vi "All Sensors.vi"() -> ()   [LabVIEW 2019]
uses:
  <vilib>/Platform/TimedLoop/XDataNode/timing_clust.ctl
  <vilib>/Platform/TimedLoop/XDataNode/nitl_modes.ctl
  <vilib>/Platform/TimedLoop/XDataNode/wakeup.ctl
  <vilib>/myRIO/Instrument Drivers/Onboard IO/I2C/typedefs/I2C User Configuration.ctl
  <vilib>/myRIO/Instrument Drivers/Onboard IO/I2C/typedefs/I2C Transfer Rate.ctl
  <vilib>/myRIO/Instrument Drivers/Onboard IO/I2C/typedefs/I2C Reference.ctl
  <vilib>/myRIO/Common/Instrument Driver Framework/Utilities/typedefs/myRIO Generic Hardware Reference.ctl
  <vilib>/myRIO/Common/Instrument Driver Framework/Utilities/typedefs/Hardware Version Enum.ctl
  <vilib>/myRIO/Common/Instrument Driver Framework/Utilities/typedefs/myRIO v1.0 Reference.ctl
  <vilib>/myRIO/Common/Instrument Driver Framework/Utilities/typedefs/Generic FPGA Reference.ctl
  <vilib>/myRIO/Common/Instrument Driver Framework/myRIO v1.0/I2C/typedefs/I2C Channels Enum.ctl
  <vilib>/myRIO/Instrument Drivers/Onboard IO/I2C/typedefs/I2C Configuration.ctl
  <vilib>/userDefined/High Color/nirio_resource_hc.ctl
  <vilib>/myRIO/Common/Instrument Driver Framework/Utilities/vis/Is FPGA Ref Available.vi
  <vilib>/myRIO/Common/Instrument Driver Framework/myRIO v1.0/I2C/vis/myRIO v1.1 Open I2C.vi
  <vilib>/myRIO/Instrument Drivers/Onboard IO/I2C/vis/Configure.vi
  <vilib>/myRIO/Instrument Drivers/Onboard IO/I2C/vis/Write.vi
  <vilib>/myRIO/Instrument Drivers/Onboard IO/I2C/vis/Write Read.vi
  <vilib>/myRIO/Common/Instrument Driver Framework/Utilities/vis/Validate Channels.vi
  <vilib>/myRIO/Common/Instrument Driver Framework/myRIO v1.0/I2C/vis/myRIO v1.0 Reserve I2C.vi
  <vilib>/myRIO/Common/Instrument Driver Framework/myRIO v1.0/I2C/vis/myRIO v1.0 Build MUX Configuration I2C.vi
  <vilib>/myRIO/Common/Instrument Driver Framework/myRIO v1.0/Resource Manager/vis/myRIO v1.0 Reserve Channel List.vi
  <vilib>/myRIO/Common/Instrument Driver Framework/myRIO v1.0/Resource Manager/vis/myRIO v1.0 Create Configuration List.vi
  <vilib>/myRIO/Common/Instrument Driver Framework/myRIO v1.0/Resource Manager/vis/myRIO v1.0 Reserve Channel.vi
  <vilib>/myRIO/Common/Instrument Driver Framework/myRIO v1.0/Resource Manager/vis/myRIO v1.0 Unreserve Channel.vi
  <vilib>/myRIO/Common/Instrument Driver Framework/myRIO v1.0/Resource Manager/vis/myRIO v1.0 Build Mutex Name.vi
  <vilib>/Utility/VariantDataType/GetNumericInfo.vi
  <vilib>/Utility/error.llb/Error Cluster From Error Code.vi
  <vilib>/myRIO/Common/Instrument Driver Framework/myRIO v1.0/myRIO v1.1 Open.vi
  <vilib>/myRIO/Common/Instrument Driver Framework/Utilities/vis/IO Manager.vi
  <vilib>/myRIO/Common/Instrument Driver Framework/Utilities/vis/Configuration Manager.vi
  <vilib>/myRIO/Common/Instrument Driver Framework/myRIO v1.0/Resource Manager/vis/myRIO v1.0 Configure IO.vi
  <vilib>/myRIO/Common/Instrument Driver Framework/myRIO v1.0/myRIO v1.0 Close.vi
  <vilib>/myRIO/Common/Instrument Driver Framework/myRIO v1.0/I2C/vis/myRIO v1.0 Configure I2C.vi
  <vilib>/myRIO/Common/Instrument Driver Framework/myRIO v1.0/I2C/vis/myRIO v1.0 Write I2C.vi
  <vilib>/myRIO/Common/Instrument Driver Framework/myRIO v1.0/I2C/vis/myRIO v1.0 Read I2C.vi
  <vilib>/platform/TimedLoop/XDataNode/XDataNode.xnode
  <vilib>/myRIO/Express VI/Onboard IO/I2C/I2C Express VI.xnode
  <vilib>/myRIO/Instrument Drivers/Onboard IO/I2C/vis/myRIO I2C Open.xnode
  <vilib>/Platform/TimedLoop/XDataNode/XDNodeRunTimeDep.lvlib
  <vilib>/myRIO/Instrument Drivers/Onboard IO/I2C/I2C.lvlib
panel:
  out "Magnetic field [G] 74-2 2":cluster{dbl, dbl, dbl}(graph) caption="Waveform Chart"
  out "Z_mag 6":dbl
  out "Y_mag 6":dbl
  out "X_mag 6":dbl
  out "Z 6":i16
  out "Y 6":i16
  out "X 6":i16
  out "DATA1 6":u8[](array[numeric]) format="%02x"
  in  "[ESC]":bool
  out "appended array":u8[](array[numeric])
  out "Magnetic field [G] 74-2":cluster{dbl, dbl, dbl}(graph) caption="Waveform Chart"
  out "Z_mag 5":dbl
  out "Y_mag 5":dbl
  out "X_mag 5":dbl
  out "Z 5":i16
  out "Y 5":i16
  out "X 5":i16
  out "DATA1 5":u8[](array[numeric]) format="%02x"
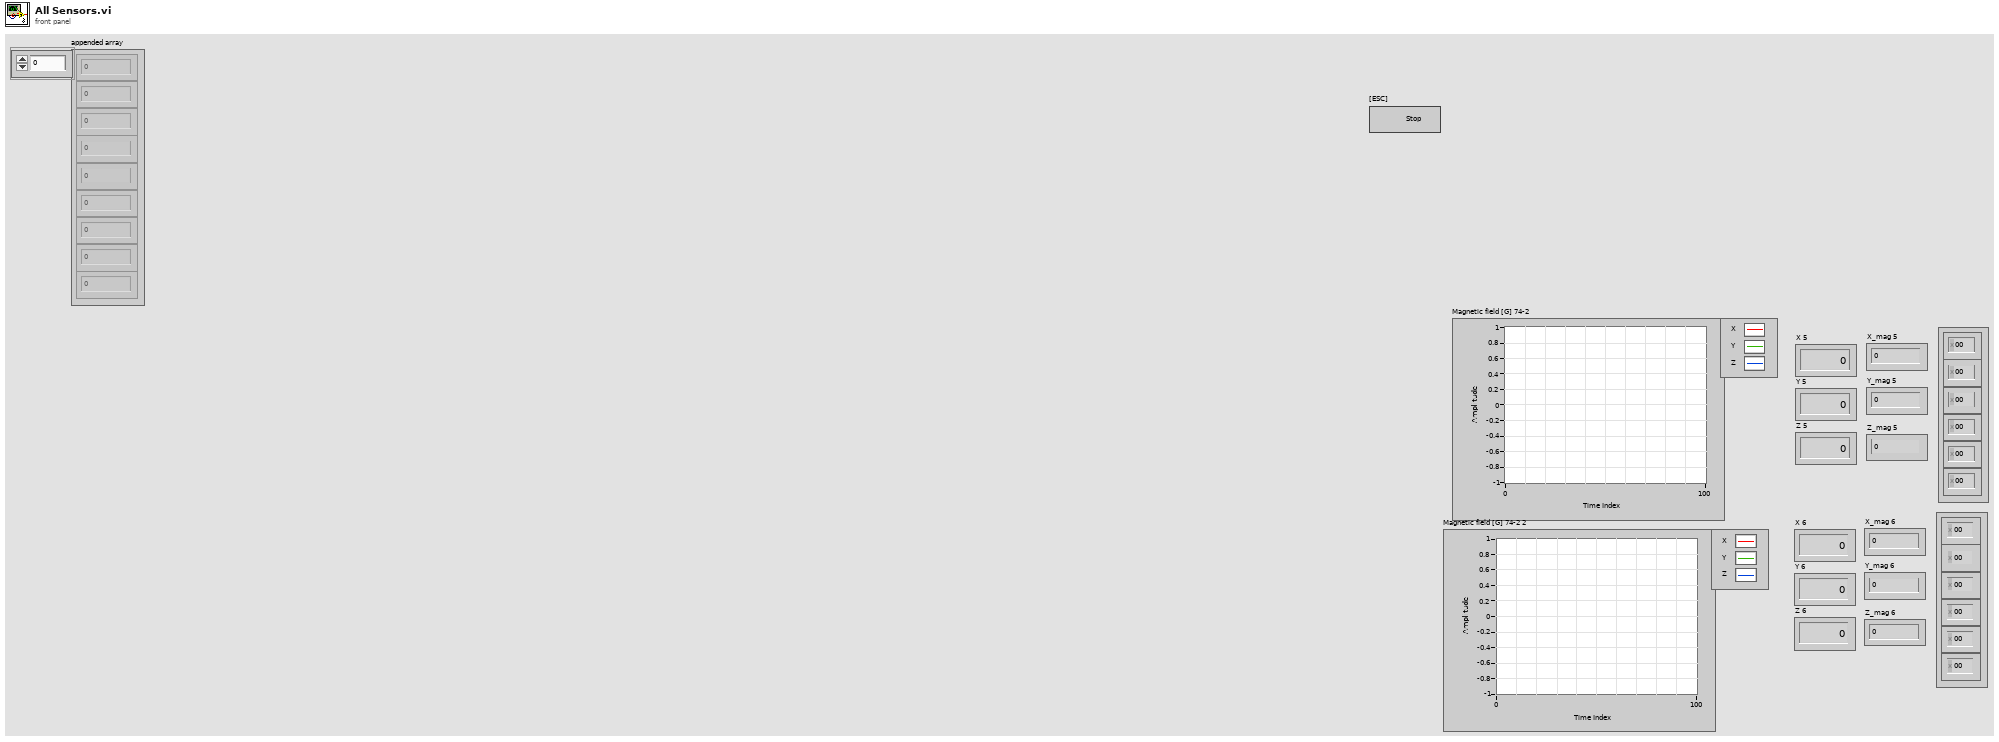
[diagram p1: front panel]
types:
  T1 = typedef "XDNodeRunTimeDep.lvlib/timing_clust.ctl" = cluster{"Expected End [f-1]":u64, "Actual End [f-1]":u64, "Finished Late? [f-1]":bool, "Expected End [i-1]":u64, "Actual End [i-1]":u64, "Finished Late? [i-1]":bool, "Expected Start [i]":u64, "Actual Start [i]":u64, "Expected Start [f]":u64, "Actual Start [f]":u64, "Source Name":string, "Structure Name":string, "Period":i64, "Deadline":i64, "Offset":i64, "Start":i64, "Priority":i32, "Timeout":i32, "Mode":T2, "Wakeup Reason":T3, "Error":errorcluster, "Source Type":string, "Secondary Source Type":string, "Global End Time":u64, "Global Start Time":u64, "Frame Duration":u64, "Iteration Duration":u64, "Assigned CPU":i32, "I/O Scan Engine Mode":u32}
  T2 = typedef "XDNodeRunTimeDep.lvlib/nitl_modes.ctl" = enum32{"No Change", "Process missed periods, maintain original phase", "Discard missed periods, maintain original phase", "Process missed periods, ignore original phase", "Discard missed periods, ignore original phase"}
  T3 = typedef "XDNodeRunTimeDep.lvlib/wakeup.ctl" = enum32{"Normal", "Aborted", "Asynchronous wakeup", "Timing source error", "Timed loop error", "Timeout"}
  T4 = typedef "I2C.lvlib/I2C Reference.ctl" = cluster{"myRIO Reference":T5, "I2C Channels Enum":T9, "I2C Configuration":T10}
  T5 = typedef "myRIO Generic Hardware Reference.ctl" = cluster{"myRIO Model":T6, "myRIO Hardware Reference":T7}
  T6 = typedef "Hardware Version Enum.ctl" = enum16{"Unknown", "myRIO-1900", "myRIO-1950", "roboRIO", "NI ELVIS RIO CM", "ELVIS III"}
  T7 = typedef "myRIO v1.0 Reference.ctl" = cluster{"Generic FPGA Reference":T8, "Allow multiple opens":bool}
  T8 = typedef "Generic FPGA Reference.ctl" = refnum<k20>
  T9 = typedef "I2C Channels Enum.ctl" = enum16{"Not Connected", "A/I2C", "B/I2C", "I2C/I2C"}
  T10 = typedef "I2C.lvlib/I2C Configuration.ctl" = cluster{"I2C Transfer Rate":T11}
  T11 = typedef "I2C.lvlib/I2C Transfer Rate.ctl" = enum16{"Standard mode (100 kbps)", "Fast mode (400 kbps)"}
  T12 = typedef "I2C.lvlib/I2C User Configuration.ctl" = cluster{"I2C Transfer Rate":T11}
  T13 = typedef "nirio_resource_hc.ctl" = tag
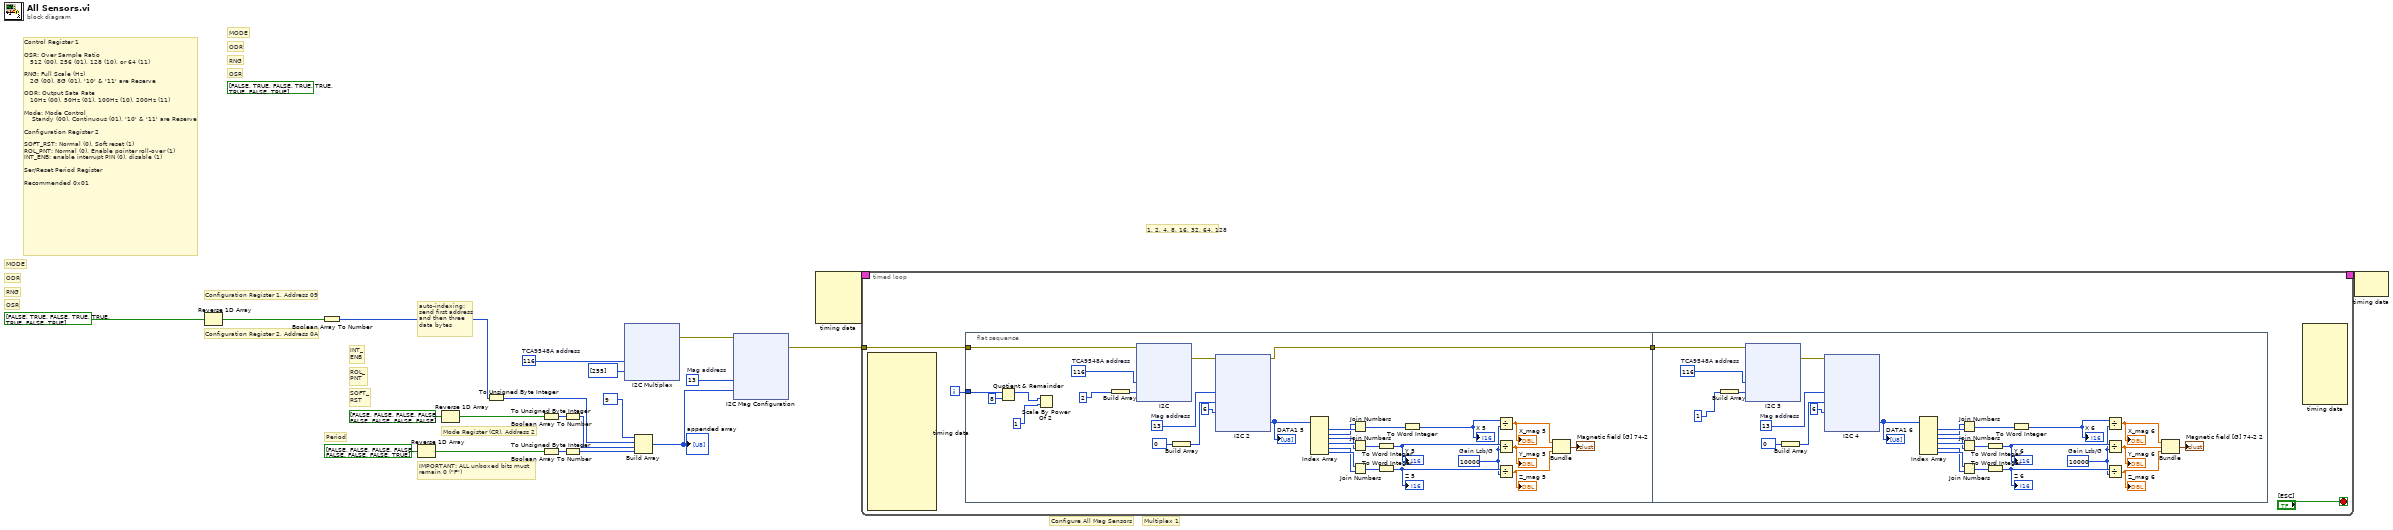
[diagram p0: block diagram]
diagram:
  (unwired) bool[] [FALSE, TRUE, FALSE, TRUE, TRUE, TRUE, FALSE, TRUE]
  w3 = u8 116  # TCA9548A address
  w2 = u8 13  # Mag address
  # "1, 2, 4, 8, 16, 32, 64, 128"
  # "ODR"
  # "MODE"
  # "RNG"
  # "OSR"
  # "Multiplex 1"
  # "INT_\nENB"
  # "ROL_\nPNT"
  # "ODR"
  # "auto-indexing:\nsend first address\nand then three\ndata bytes"
  # "Control Register 1\n\nOSR: Over Sample Ratio \n   512 (00), 256 (01), 128 (10), or 64 (11)\n\nRNG: Full Scale (Hz)\n   2G (00), 8G (01), '10' & '11' are Reserve\n\nODR: Output Sata Rate\n   10Hz (00), 50Hz (01), 100Hz (10), 200Hz (11)\n\nMode: Mode Control\n    Standy (00), Continuous (01), '10' & '11' are Reserve     \n\nConfiguration Register 2\n\nSOFT_RST: Normal (0), Soft reset (1)\nROL_PNT: Normal (0), Enable pointer roll-over (1)\nINT_ENB: enable interrupt PIN (0), disable (1)\n\nSer/Reset Period Register\n\nRecommended 0x01"
  # "IMPORTANT: ALL unboxed bits must\nremain 0 (\"F\")"
  # "Configure All Mag Sensors"
  # "Period"
  # "Mode Register (CR), Address 2"
  # "Configuration Register 2, Address 0A"
  # "SOFT_\nRST"
  # "Configuration Register 1, Address 09"
  # "MODE"
  # "RNG"
  # "OSR"
  n1 = Reverse 1D Array(array=bool[] [FALSE, TRUE, FALSE, TRUE, TRUE, TRUE, FALSE, TRUE]) -> (reversed array=w18:bool[])
  n2 = Boolean Array To Number(Boolean array=w18) -> (number=w12:u32)
  n3 = Reverse 1D Array(array=bool[] [FALSE, FALSE, FALSE, FALSE, FALSE, FALSE, FALSE, TRUE]) -> (reversed array=w15:bool[])
  n4 = Reverse 1D Array(array=bool[] [FALSE, FALSE, FALSE, FALSE, FALSE, FALSE, FALSE, FALSE]) -> (reversed array=w17:bool[])
  n5 = To Unsigned Byte Integer(number=w12) -> (unsigned 8bit integer=w9:u8)
  n6 = Boolean Array To Number(Boolean array=w17) -> (number=w11:u32)
  n7 = Boolean Array To Number(Boolean array=w15) -> (number=w10:u32)
  n8 = To Unsigned Byte Integer(number=w11) -> (unsigned 8bit integer=w7:u8)
  n9 = To Unsigned Byte Integer(number=w10) -> (unsigned 8bit integer=w6:u8)
  n10 = xnode "I2C Multiplex"("Slave Address (7-bit)"=w3, "Bytes to Write"=u8[] [255]) -> ("error out"=w4:errorcluster)  [unwired: 1 in]
  n11 = Build Array "Build Array"(u8 9 ("address"), w9, w7, w6) -> (w8:u8[])
  "appended array" <- w8
  n12 = xnode "I2C Mag Configuration"("Slave Address (7-bit)"=w2, "Bytes to Write"=w8, "error in (no error)"=w4) -> ("error out"=w1:errorcluster)
  n13 = node-c288() -> (w21:T1)  [unwired: 4 in]
  n14 = timed-loop {
    timing: w21 -> [_]
    timing-out: [_] -> w20
    tunnel: w1 -> [w24]
    i -> [w25]
    stop <- "[ESC]" stop-if-true
    n15 = node-c288() -> ()  [unwired: 1 in, 17 out]
    n16 = flat-sequence {
      tunnel: w25 -> [w52]
      tunnel: w24 -> [w30]
      tunnel: [w27] -> w22
      tunnel: w22 -> [w136]
      frame #0 {
        w32 = u8 116  # TCA9548A address
        w33 = u8 13  # Mag address
        w45 = i16 10000  # Gain Lsb/G
        n17 = Quotient & Remainder(x=w52, y=8) -> (x-y*floor(x/y)=w29:i32)  [unwired: 1 out]
        n18 = Scale By Power Of 2(n=w29, x=1) -> ()  [unwired: 1 out]
        n19 = Build Array(2) -> (w31:i32[])
        n20 = xnode "I2C"("Slave Address (7-bit)"=w32, "Bytes to Write"=w31, "error in (no error)"=w30) -> ("error out"=w57:errorcluster)
        n21 = Build Array(u8 0) -> (w54:u8[])
        n22 = xnode "I2C 2"("Slave Address (7-bit)"=w33, "Bytes to Write"=w54, "Byte Count"=u32 6, "error in (no error)"=w57) -> ("Bytes Read"=w34:u8[], "error out"=w27:errorcluster)
        "DATA1 5" <- w34
        n23 = Index Array "Index Array"(array=w34) -> (element #1=w41:u8, element #2=w40:u8, element #3=w38:u8, element #4=w39:u8, element #5=w36:u8, element #6=w37:u8)  [unwired: 6 in]
        n24 = Join Numbers(hi=w40, lo=w41) -> ((hi.lo)=w51:u16)
        n25 = Join Numbers(hi=w39, lo=w38) -> ((hi.lo)=w49:u16)
        n26 = Join Numbers(hi=w37, lo=w36) -> ((hi.lo)=w50:u16)
        n27 = To Word Integer(number=w49) -> (16bit integer=w47:i16)
        "Y 5" <- w47
        n28 = To Word Integer(number=w50) -> (16bit integer=w46:i16)
        "Z 5" <- w46
        n29 = To Word Integer(number=w51) -> (16bit integer=w48:i16)
        "X 5" <- w48
        n30 = Divide(x=w48, y=w45) -> (x/y=w44:dbl)
        "X_mag 5" <- w44
        n31 = Divide(x=w47, y=w45) -> (x/y=w43:dbl)
        "Y_mag 5" <- w43
        n32 = Divide(x=w46, y=w45) -> (x/y=w42:dbl)
        "Z_mag 5" <- w42
        n33 = Bundle(w44, w43, w42) -> (→"Magnetic field [G] 74-2":cluster{dbl, dbl, dbl})  [unwired: 1 in]
      }
      frame #1 {
        w139 = u8 116  # TCA9548A address
        w140 = u8 13  # Mag address
        w152 = i16 10000  # Gain Lsb/G
        n34 = Build Array(1) -> (w138:i32[])
        n35 = xnode "I2C 3"("Slave Address (7-bit)"=w139, "Bytes to Write"=w138, "error in (no error)"=w136) -> ("error out"=w162:errorcluster)
        n36 = Build Array(u8 0) -> (w159:u8[])
        n37 = xnode "I2C 4"("Slave Address (7-bit)"=w140, "Bytes to Write"=w159, "Byte Count"=u32 6, "error in (no error)"=w162) -> ("Bytes Read"=w141:u8[])  [unwired: 1 out]
        "DATA1 6" <- w141
        n38 = Index Array "Index Array"(array=w141) -> (element #1=w148:u8, element #2=w147:u8, element #3=w145:u8, element #4=w146:u8, element #5=w143:u8, element #6=w144:u8)  [unwired: 6 in]
        n39 = Join Numbers(hi=w147, lo=w148) -> ((hi.lo)=w158:u16)
        n40 = Join Numbers(hi=w146, lo=w145) -> ((hi.lo)=w156:u16)
        n41 = Join Numbers(hi=w144, lo=w143) -> ((hi.lo)=w157:u16)
        n42 = To Word Integer(number=w156) -> (16bit integer=w154:i16)
        "Y 6" <- w154
        n43 = To Word Integer(number=w157) -> (16bit integer=w153:i16)
        "Z 6" <- w153
        n44 = To Word Integer(number=w158) -> (16bit integer=w155:i16)
        "X 6" <- w155
        n45 = Divide(x=w155, y=w152) -> (x/y=w151:dbl)
        "X_mag 6" <- w151
        n46 = Divide(x=w154, y=w152) -> (x/y=w150:dbl)
        "Y_mag 6" <- w150
        n47 = Divide(x=w153, y=w152) -> (x/y=w149:dbl)
        "Z_mag 6" <- w149
        n48 = Bundle(w151, w150, w149) -> (→"Magnetic field [G] 74-2 2":cluster{dbl, dbl, dbl})  [unwired: 1 in]
      }
    }
    n49 = node-c288() -> ()  [unwired: 8 in, 1 out]
  }
  n50 = node-c288(w20) -> ()  [unwired: 1 out]
